vi "Get Variant Name.vi"(8 "error in":errorcluster, 11 "Variant_in":variant) -> (0 "error out":errorcluster, 1 "found":bool, 2 "Name":string, 3 "Variant_out":variant)   [LabVIEW 2021, in "DataTypes_CIF_U.lvlib"]
doc: "This will get an attribute of \"Name\" on a variant."
uses:
  DataTypes_CIF_U.lvlib
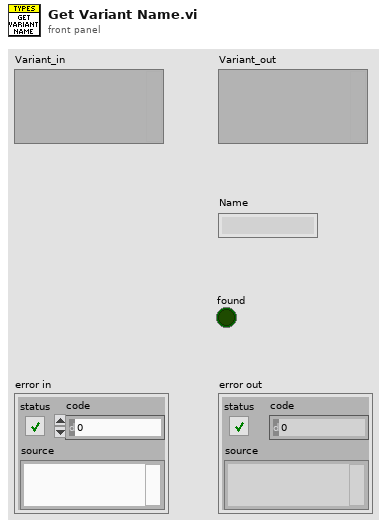
[diagram p1: front panel]
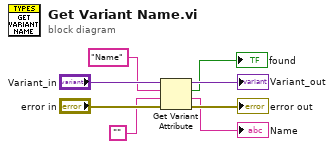
[diagram p0: block diagram]
diagram:
  n1 = Get Variant Attribute(Variant="Variant_in", name="Name", default value (empty Variant)="", error in="error in") -> (duplicate Variant=→"Variant_out":variant, found=→"found":bool, value=→"Name":string, error out=→"error out":errorcluster)
